vi "Finish.vi"   [LabVIEW 2013]
doc: "This VI is called just before exiting. It is expected to close I/O refnum, save collected data, etc."
uses:
  <vilib>/Rock Robotics/WPI/Joystick/WPI_JoystickGetSetRefNum.vi
  <vilib>/Rock Robotics/WPI/RobotDrive/WPI_RobotDriveGetSetRefNum.vi
types:
  T1 = typedef "WPI_SolenoidDevRef.ctl" = cluster{"DevStatus":errorcluster, "Solenoid Module":T2, "Forward Solenoid Channel":T3, "Reverse Solenoid Channel":T3}
  T2 = typedef "FPGA_TypedefSolenoidModule.ctl" = enum16{"Solenoid Module 1", "Solenoid Module 2"}
  T3 = typedef "WPI_SolenoidChannel.ctl" = enum8{"Solenoid 1", "Solenoid 2", "Solenoid 3", "Solenoid 4", "Solenoid 5", "Solenoid 6", "Solenoid 7", "Solenoid 8", "Invalid"}
  T4 = typedef "WPI_DigitalInputDevRef.ctl" = cluster{"DevStatus":errorcluster, "DIO Channel":T5, "Digital Module":T6}
  T5 = typedef "FPGA_DIOChannel.ctl" = enum8{"DIO 1", "DIO 2", "DIO 3", "DIO 4", "DIO 5", "DIO 6", "DIO 7", "DIO 8", "DIO 9", "DIO 10", "DIO 11", "DIO 12", "DIO 13", "DIO 14", "Invalid"}
  T6 = typedef "FPGA_TypedefDigitalModule.ctl" = enum16{"Digital Module 1", "Digital Module 2"}
  T7 = typedef "WPI_JoystickDevRef.ctl" = cluster{"Device":T8}
  T8 = typedef "WPI_JoystickDeviceEnum.ctl" = enum16{"USB 1", "USB 2", "USB 3", "USB 4", "Kinect 1", "Kinect 2"}
  T9 = typedef "WPI_RobotDriveDevRef.ctl" = cluster{"DevStatus":errorcluster, "Motors[]":T10[], "Square Inputs":bool, "Max Output":dbl, "Isochronous":bool}
  T10 = typedef "WPI_MotorControlDeviceRef.ctl" = cluster{"DeviceStatus":errorcluster, "Type":enum16{"PWM", "CAN"}, "PWM":cluster{"Digital Module":T6, "PWM Channel":T11, "DeadBand":T12}, "CAN":cluster{"Device Number":u8, "Control Mode":T13, "Semaphore":T14, "Max Vout":dbl}, "Invert":bool, "TransformRef":T15, "InvTransformRef":T15}
  T11 = typedef "FPGA_DIOPWMChannel.ctl" = enum8{"PWM 1", "PWM 2", "PWM 3", "PWM 4", "PWM 5", "PWM 6", "PWM 7", "PWM 8", "PWM 9", "PWM 10", "Invalid"}
  T12 = typedef "WPI_PWMDeadband.ctl" = cluster{"Name":string, "maxPositivePwm":i32, "minPositivePwm":i32, "centerPwm":i32, "maxNegativePwm":i32, "minNegativePwm":i32, "angularRange":u16}
  T13 = typedef "WPI_CANJaguar_ControlMode.ctl" = enum8{"Percent VBus", "Current", "Speed", "Position", "Voltage"}
  T14 = typedef "Semaphore RefNum" = refnum<k1>
  T15 = typedef "WPI_PWMTransform_ConPane.ctl" = refnum<vi>
  T16 = typedef "WPI_RelayDevRef.ctl" = cluster{"DevStatus":errorcluster, "Relay Channel":T17, "Digital Module":T6, "Relay Direction":T18}
  T17 = typedef "FPGA_DIORelayChannel.ctl" = enum8{"Relay 1", "Relay 2", "Relay 3", "Relay 4", "Relay 5", "Relay 6", "Relay 7", "Relay 8", "Invalid"}
  T18 = typedef "WPI_RelayDirection.ctl" = enum16{"Both directions", "Forward only", "Reverse only"}
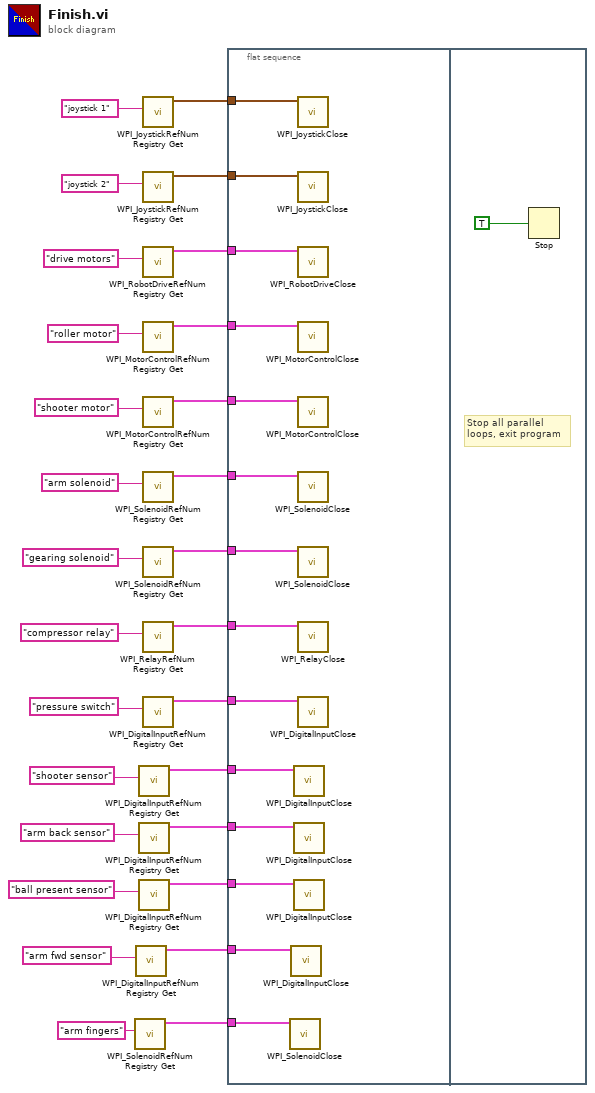
[diagram p0: block diagram]
diagram:
  n1 = call <vilib>:"WPI_SolenoidRefNum Registry Get.vi"("refnum name"="arm fingers") -> ("SolenoidDevRef"=w1:T1)  [unwired: 9 in, 1 out]
  n2 = call <vilib>:"WPI_DigitalInputRefNum Registry Get.vi"("refnum name"="arm fwd sensor") -> ("DigitalInputDevRef"=w4:T4)  [unwired: 9 in, 1 out]
  n3 = call <vilib>:"WPI_DigitalInputRefNum Registry Get.vi"("refnum name"="shooter sensor") -> ("DigitalInputDevRef"=w9:T4)  [unwired: 9 in, 1 out]
  n4 = call <vilib>:"WPI_DigitalInputRefNum Registry Get.vi"("refnum name"="arm back sensor") -> ("DigitalInputDevRef"=w8:T4)  [unwired: 9 in, 1 out]
  n5 = call <vilib>:"WPI_DigitalInputRefNum Registry Get.vi"("refnum name"="ball present sensor") -> ("DigitalInputDevRef"=w5:T4)  [unwired: 9 in, 1 out]
  n6 = call <vilib>:"WPI_JoystickRefNum Registry Get.vi"("refnum name"="joystick 1") -> ("JoystickDevRef"=w25:T7)  [unwired: 1 in, 9 out]
  n7 = call <vilib>:"WPI_JoystickRefNum Registry Get.vi"("refnum name"="joystick 2") -> ("JoystickDevRef"=w12:T7)  [unwired: 1 in, 9 out]
  n8 = call <vilib>:"WPI_RobotDriveRefNum Registry Get.vi"("refnum name"="drive motors") -> ("RobotDriveDevRef"=w26:T9)  [unwired: 1 in, 9 out]
  n9 = call <vilib>:"WPI_MotorControlRefNum Registry Get.vi"("refnum name"="roller motor") -> ("MotorControlDevRef"=w24:T10)  [unwired: 9 in, 1 out]
  n10 = call <vilib>:"WPI_MotorControlRefNum Registry Get.vi"("refnum name"="shooter motor") -> ("MotorControlDevRef"=w23:T10)  [unwired: 9 in, 1 out]
  n11 = call <vilib>:"WPI_SolenoidRefNum Registry Get.vi"("refnum name"="arm solenoid") -> ("SolenoidDevRef"=w20:T1)  [unwired: 9 in, 1 out]
  n12 = call <vilib>:"WPI_SolenoidRefNum Registry Get.vi"("refnum name"="gearing solenoid") -> ("SolenoidDevRef"=w13:T1)  [unwired: 9 in, 1 out]
  n13 = call <vilib>:"WPI_RelayRefNum Registry Get.vi"("refnum name"="compressor relay") -> ("RelayDevRef"=w18:T16)  [unwired: 9 in, 1 out]
  n14 = call <vilib>:"WPI_DigitalInputRefNum Registry Get.vi"("refnum name"="pressure switch") -> ("DigitalInputDevRef"=w17:T4)  [unwired: 9 in, 1 out]
  n15 = flat-sequence {
    tunnel: w26 -> [w42]
    tunnel: w25 -> [w41]
    tunnel: w24 -> [w40]
    tunnel: w23 -> [w39]
    tunnel: w20 -> [w38]
    tunnel: w18 -> [w37]
    tunnel: w17 -> [w36]
    tunnel: w13 -> [w35]
    tunnel: w12 -> [w34]
    tunnel: w9 -> [w33]
    tunnel: w8 -> [w32]
    tunnel: w5 -> [w31]
    tunnel: w4 -> [w30]
    tunnel: w1 -> [w29]
    frame #0 {
      n16 = call <vilib>:"WPI_SolenoidClose.vi"("SolenoidDevRef"=w29) -> ()  [unwired: 10 in, 1 out]
      n17 = call <vilib>:"WPI_DigitalInputClose.vi"("DigitalInputDevRef"=w30) -> ()  [unwired: 10 in, 1 out]
      n18 = call <vilib>:"WPI_DigitalInputClose.vi"("DigitalInputDevRef"=w33) -> ()  [unwired: 10 in, 1 out]
      n19 = call <vilib>:"WPI_DigitalInputClose.vi"("DigitalInputDevRef"=w32) -> ()  [unwired: 10 in, 1 out]
      n20 = call <vilib>:"WPI_DigitalInputClose.vi"("DigitalInputDevRef"=w31) -> ()  [unwired: 10 in, 1 out]
      n21 = call <vilib>:"WPI_JoystickClose.vi"("JoystickDevRef"=w41) -> ()  [unwired: 11 out]
      n22 = call <vilib>:"WPI_JoystickClose.vi"("JoystickDevRef"=w34) -> ()  [unwired: 11 out]
      n23 = call <vilib>:"WPI_RobotDriveClose.vi"("RobotDriveDevRef"=w42) -> ()  [unwired: 1 in, 10 out]
      n24 = call <vilib>:"WPI_MotorControlClose.vi"("MotorControlDevRef"=w40) -> ()  [unwired: 10 in, 1 out]
      n25 = call <vilib>:"WPI_MotorControlClose.vi"("MotorControlDevRef"=w39) -> ()  [unwired: 10 in, 1 out]
      n26 = call <vilib>:"WPI_SolenoidClose.vi"("SolenoidDevRef"=w38) -> ()  [unwired: 10 in, 1 out]
      n27 = call <vilib>:"WPI_SolenoidClose.vi"("SolenoidDevRef"=w35) -> ()  [unwired: 10 in, 1 out]
      n28 = call <vilib>:"WPI_RelayClose.vi"("RelayDevRef"=w37) -> ()  [unwired: 10 in, 1 out]
      n29 = call <vilib>:"WPI_DigitalInputClose.vi"("DigitalInputDevRef"=w36) -> ()  [unwired: 10 in, 1 out]
    }
    frame #1 {
      # "Stop all parallel\nloops, exit program"
      n30 = Stop(stop? (T)=TRUE ("Quit")) -> ()
    }
  }
